vi "ScriptCommands.vi"(11 "Auton Routines":T1[](array[typedef])) -> ()   [LabVIEW 2013]
uses:
  Command Type.ctl
  <vilib>/Rock Robotics/WPI/DriverStation/DriverStationLCD/WPI_DriverStationLCDLCDLine.ctl
  Intake Actions.ctl
  <vilib>/Rock Robotics/WPI/RobotDrive/WPI_RobotDriveGetSetRefNum.vi
  Auto Pickup Global.vi
  Robot Global Data.vi
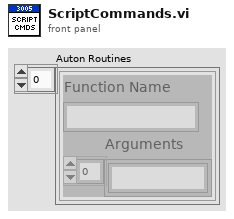
[diagram p1: front panel]
types:
  T1 = typedef "Command Type.ctl" = cluster{"Function Name":string, "Arguments":string[]}
  T2 = typedef "WPI_DriverStationLCDLCDLine.ctl" = enum16{"Main - Line 1", "User - Line 2", "User - Line 3", "User - Line 4", "User - Line 5", "User - Line 6"}
  T3 = typedef "Intake Actions.ctl" = enum16{"Extend", "Contain", "Motor Still", "Motor Outward", "Motor Inward", "Collect", "Pass", "Herd", "Contain Off", "Collect Delay Off", "Patea"}
  T4 = typedef "WPI_EncoderDevRef.ctl" = cluster{"DevStatus":errorcluster, "EncoderIndex":T5, "CounterIndex":T6, "DistancePerCount":dbl, "Decoding Type":T7}
  T5 = typedef "FPGA_EncoderIdx.ctl" = enum8{"Enc 0", "Enc 1", "Enc 2", "Enc 3", "Invalid"}
  T6 = typedef "FPGA_CounterCtrSystemIndex.ctl" = enum8{"Ctr 0", "Ctr 1", "Ctr 2", "Ctr 3", "Ctr 4", "Ctr 5", "Ctr 6", "Ctr 7", "Invalid"}
  T7 = typedef "WPI_EncoderType.ctl" = enum16{"1x", "2x", "4x"}
  T8 = typedef "WPI_RobotDriveDevRef.ctl" = cluster{"DevStatus":errorcluster, "Motors[]":T9[], "Square Inputs":bool, "Max Output":dbl, "Isochronous":bool}
  T9 = typedef "WPI_MotorControlDeviceRef.ctl" = cluster{"DeviceStatus":errorcluster, "Type":enum16{"PWM", "CAN"}, "PWM":cluster{"Digital Module":T10, "PWM Channel":T11, "DeadBand":T12}, "CAN":cluster{"Device Number":u8, "Control Mode":T13, "Semaphore":T14, "Max Vout":dbl}, "Invert":bool, "TransformRef":T15, "InvTransformRef":T15}
  T10 = typedef "FPGA_TypedefDigitalModule.ctl" = enum16{"Digital Module 1", "Digital Module 2"}
  T11 = typedef "FPGA_DIOPWMChannel.ctl" = enum8{"PWM 1", "PWM 2", "PWM 3", "PWM 4", "PWM 5", "PWM 6", "PWM 7", "PWM 8", "PWM 9", "PWM 10", "Invalid"}
  T12 = typedef "WPI_PWMDeadband.ctl" = cluster{"Name":string, "maxPositivePwm":i32, "minPositivePwm":i32, "centerPwm":i32, "maxNegativePwm":i32, "minNegativePwm":i32, "angularRange":u16}
  T13 = typedef "WPI_CANJaguar_ControlMode.ctl" = enum8{"Percent VBus", "Current", "Speed", "Position", "Voltage"}
  T14 = typedef "Semaphore RefNum" = refnum<k1>
  T15 = typedef "WPI_PWMTransform_ConPane.ctl" = refnum<vi>
  T16 = typedef "WPI_CounterDevRef.ctl" = cluster{"DevStatus":errorcluster, "CntIndex":T6}
  T17 = typedef "WPI_GyroDevRef.ctl" = cluster{"DevStatus":errorcluster, "Analog Module":T18, "Analog Channel":T19, "Offset":dbl, "Gain (VoltsPerDegree/Second)":dbl}
  T18 = typedef "FPGA_TypedefAnalogModule.ctl" = enum16{"Analog Module 1", "Analog Module 2"}
  T19 = typedef "FPGA_AIChannel.ctl" = enum8{"AI 1", "AI 2", "AI 3", "AI 4", "AI 5", "AI 6", "AI 7", "AI 8", "Invalid"}
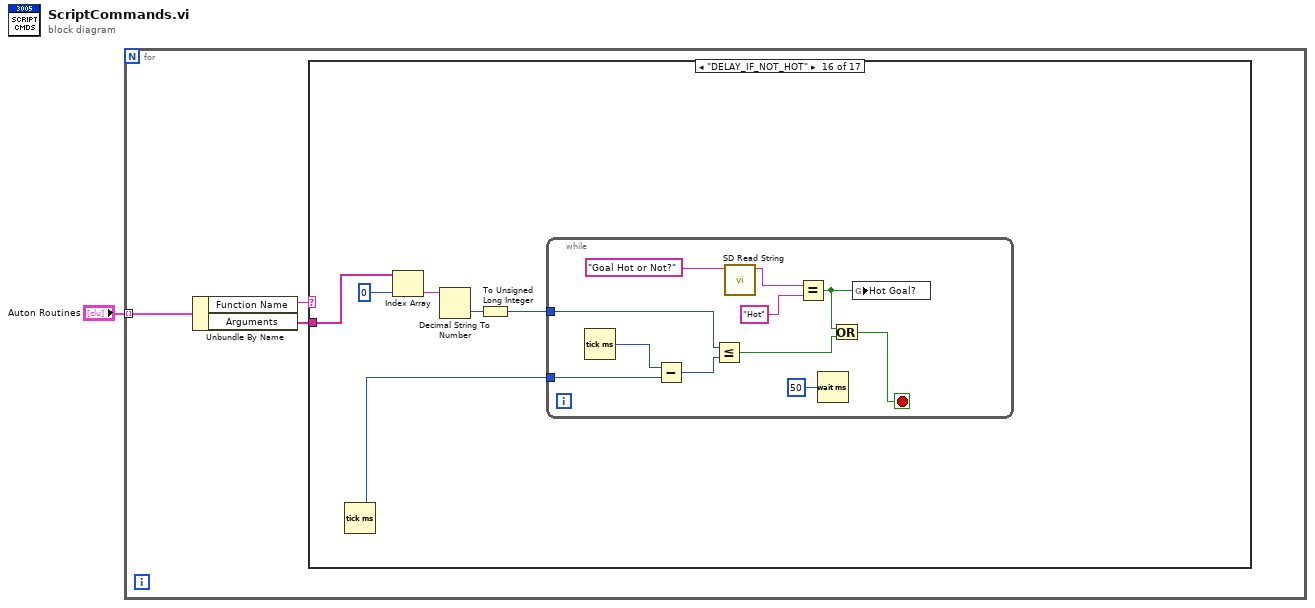
[diagram p0: block diagram]
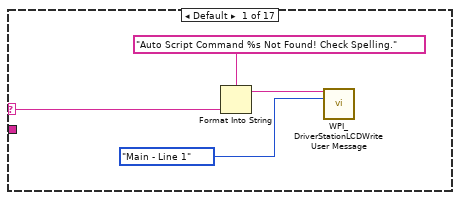
[diagram p2: hidden frame]
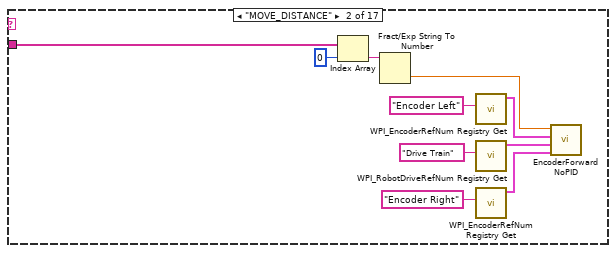
[diagram p3: hidden frame]
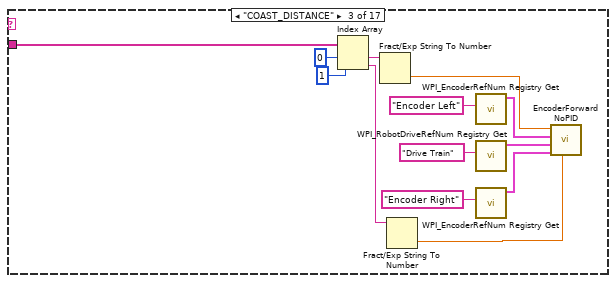
[diagram p4: hidden frame]
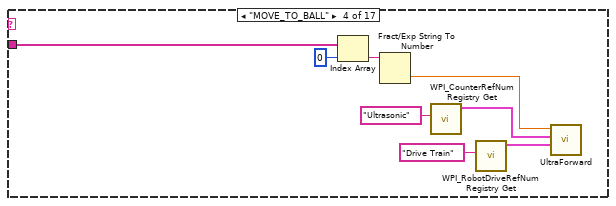
[diagram p5: hidden frame]
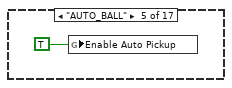
[diagram p6: hidden frame]
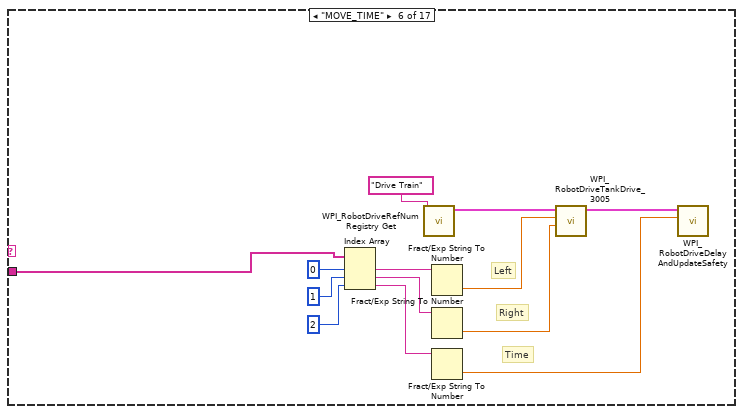
[diagram p7: hidden frame]
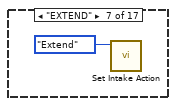
[diagram p8: hidden frame]
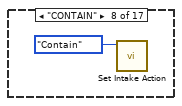
[diagram p9: hidden frame]
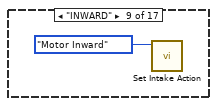
[diagram p10: hidden frame]
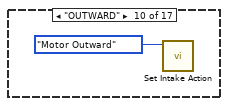
[diagram p11: hidden frame]
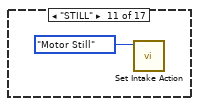
[diagram p12: hidden frame]
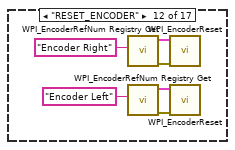
[diagram p13: hidden frame]
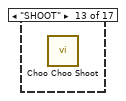
[diagram p14: hidden frame]
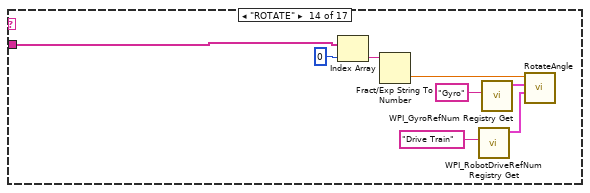
[diagram p15: hidden frame]
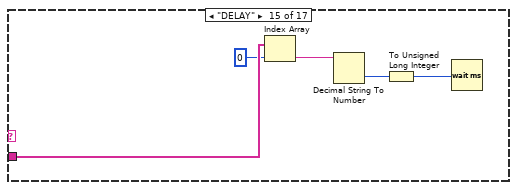
[diagram p16: hidden frame]
diagram:
  n1 = for {
    tunnel: "Auton Routines" -> [w4] mode=indexing
    n2 = Unbundle By Name(w4) -> ("Function Name"=w3:string, "Arguments"=w2:string[])
    n3 = case shown="\"DELAY_IF_NOT_HOT\"" w3 {
      selector: w3 -> [w8 _ _ _ _ _ _ _ _ _ _ _ _ _ _ _ _]
      tunnel: w2 -> [_ w18 w31 w39 _ w41 _ _ _ _ _ _ _ w72 w77 w80 _]
      frame Default {
        n4 = Format Into String(format string="Auto Script Command %s Not Found! Check Spelling.", w8) -> (resulting string=w6:string)  [unwired: 2 in, 1 out]
        n5 = call <vilib>:"WPI_DriverStationLCDWrite User Message.vi"("line text"=w6, "line"=WPI_DriverStationLCDLCDLine."Main - Line 1") -> ()  [unwired: 13 in, 1 out]
      }
      frame "MOVE_DISTANCE" {
        n6 = Index Array(array=w18, index=0) -> (element=w16:string)
        n7 = Fract/Exp String To Number(string=w16) -> (number=w9:dbl)  [unwired: 3 in, 1 out]
        n8 = call <vilib>:"WPI_EncoderRefNum Registry Get.vi"("refnum name"="Encoder Left") -> ("EncoderDevRef"=w10:T4)  [unwired: 9 in, 1 out]
        n9 = call <vilib>:"WPI_RobotDriveRefNum Registry Get.vi"("refnum name"="Drive Train") -> ("RobotDriveDevRef"=w14:T8)  [unwired: 1 in, 9 out]
        n10 = call <vilib>:"WPI_EncoderRefNum Registry Get.vi"("refnum name"="Encoder Right") -> ("EncoderDevRef"=w11:T4)  [unwired: 9 in, 1 out]
        n11 = call "EncoderForwardNoPID.vi"("EncoderDevRef 4"=w11, "RobotDriveDevRef"=w14, "EncoderDevRef"=w10, "Target"=w9) -> ()  [unwired: 5 in, 3 out]
      }
      frame "COAST_DISTANCE" {
        n12 = Index Array(array=w31, index #1=0 ("index"), index #2=1 ("index")) -> (element #1=w29:string, element #2=w20:string)
        n13 = Fract/Exp String To Number(string=w29) -> (number=w22:dbl)  [unwired: 3 in, 1 out]
        n14 = Fract/Exp String To Number(string=w20) -> (number=w21:dbl)  [unwired: 3 in, 1 out]
        n15 = call <vilib>:"WPI_EncoderRefNum Registry Get.vi"("refnum name"="Encoder Left") -> ("EncoderDevRef"=w23:T4)  [unwired: 9 in, 1 out]
        n16 = call <vilib>:"WPI_RobotDriveRefNum Registry Get.vi"("refnum name"="Drive Train") -> ("RobotDriveDevRef"=w27:T8)  [unwired: 1 in, 9 out]
        n17 = call <vilib>:"WPI_EncoderRefNum Registry Get.vi"("refnum name"="Encoder Right") -> ("EncoderDevRef"=w24:T4)  [unwired: 9 in, 1 out]
        n18 = call "EncoderForwardNoPID.vi"("Right axis value"=w21, "EncoderDevRef 4"=w24, "RobotDriveDevRef"=w27, "EncoderDevRef"=w23, "Target"=w22) -> ()  [unwired: 4 in, 3 out]
      }
      frame "MOVE_TO_BALL" {
        n19 = Index Array(array=w39, index=0) -> (element=w37:string)
        n20 = Fract/Exp String To Number(string=w37) -> (number=w34:dbl)  [unwired: 3 in, 1 out]
        n21 = call <vilib>:"WPI_CounterRefNum Registry Get.vi"("refnum name"="Ultrasonic") -> ("CounterDevRef"=w33:T16)  [unwired: 9 in, 1 out]
        n22 = call <vilib>:"WPI_RobotDriveRefNum Registry Get.vi"("refnum name"="Drive Train") -> ("RobotDriveDevRef"=w35:T8)  [unwired: 1 in, 9 out]
        n23 = call "UltraForward.vi"("RobotDriveDevRef"=w35, "CounterDevRef in"=w33, "Target"=w34) -> ()  [unwired: 8 in, 1 out]
      }
      frame "AUTO_BALL" {
        n24 = global write "Auto Pickup Global.vi" "Enable Auto Pickup"(TRUE ("Enable Auto Pickup")) -> ()
      }
      frame "MOVE_TIME" {
        # "Time"
        # "Right"
        # "Left"
        n25 = Index Array(array=w41, index #1=0 ("index"), index #2=1 ("index"), index #3=2 ("index")) -> (element #1=w47:string, element #2=w46:string, element #3=w45:string)
        n26 = call <vilib>:"WPI_RobotDriveRefNum Registry Get.vi"("refnum name"="Drive Train") -> ("RobotDriveDevRef"=w51:T8)  [unwired: 1 in, 9 out]
        n27 = Fract/Exp String To Number(string=w47) -> (number=w44:dbl)  [unwired: 3 in, 1 out]
        n28 = Fract/Exp String To Number(string=w46) -> (number=w43:dbl)  [unwired: 3 in, 1 out]
        n29 = Fract/Exp String To Number(string=w45) -> (number=w42:dbl)  [unwired: 3 in, 1 out]
        n30 = call <vilib>:"WPI_RobotDriveTankDrive_3005.vi"("Right axis value"=w43, "Left axis value"=w44, "RobotDriveDevRef"=w51) -> ("RobotDriveDevRef"=w53:T8)  [unwired: 6 in, 2 out]
        n31 = call <vilib>:"WPI_RobotDriveDelayAndUpdateSafety.vi"("Delay (s)"=w42, "RobotDriveDevRef"=w53) -> ()  [unwired: 8 in, 2 out]
      }
      frame "EXTEND" {
        n32 = call "Set Intake Action.vi"("Action"=Intake_Actions."Extend") -> ()  [unwired: 10 in, 1 out]
      }
      frame "CONTAIN" {
        n33 = call "Set Intake Action.vi"("Action"=Intake_Actions."Contain") -> ()  [unwired: 10 in, 1 out]
      }
      frame "INWARD" {
        n34 = call "Set Intake Action.vi"("Action"=Intake_Actions."Motor Inward") -> ()  [unwired: 10 in, 1 out]
      }
      frame "OUTWARD" {
        n35 = call "Set Intake Action.vi"("Action"=Intake_Actions."Motor Outward") -> ()  [unwired: 10 in, 1 out]
      }
      frame "STILL" {
        n36 = call "Set Intake Action.vi"("Action"=Intake_Actions."Motor Still") -> ()  [unwired: 10 in, 1 out]
      }
      frame "RESET_ENCODER" {
        n37 = call <vilib>:"WPI_EncoderRefNum Registry Get.vi"("refnum name"="Encoder Right") -> ("error out"=w64:errorcluster, "EncoderDevRef"=w63:T4)  [unwired: 9 in]
        n38 = call <vilib>:"WPI_EncoderRefNum Registry Get.vi"("refnum name"="Encoder Left") -> ("error out"=w59:errorcluster, "EncoderDevRef"=w60:T4)  [unwired: 9 in]
        n39 = call <vilib>:"WPI_EncoderReset.vi"("error in (no error)"=w64, "EncoderDevRef"=w63) -> ()  [unwired: 8 in, 2 out]
        n40 = call <vilib>:"WPI_EncoderReset.vi"("error in (no error)"=w59, "EncoderDevRef"=w60) -> ()  [unwired: 8 in, 2 out]
      }
      frame "SHOOT" {
        n41 = call "Choo Choo Shoot.vi"() -> ()  [unwired: 11 in, 1 out]
      }
      frame "ROTATE" {
        n42 = Index Array(array=w72, index=0) -> (element=w70:string)
        n43 = Fract/Exp String To Number(string=w70) -> (number=w65:dbl)  [unwired: 3 in, 1 out]
        n44 = call <vilib>:"WPI_RobotDriveRefNum Registry Get.vi"("refnum name"="Drive Train") -> ("RobotDriveDevRef"=w66:T8)  [unwired: 1 in, 9 out]
        n45 = call <vilib>:"WPI_GyroRefNum Registry Get.vi"("refnum name"="Gyro") -> ("GyroDevRef"=w69:T17)  [unwired: 9 in, 1 out]
        n46 = call "RotateAngle.vi"("RobotDriveDevRef"=w66, "GyroDevRef"=w69, "Target"=w65) -> ()  [unwired: 7 in, 2 out]
      }
      frame "DELAY" {
        n47 = Index Array(array=w77, index=0) -> (element=w75:string)
        n48 = Decimal String To Number(string=w75) -> (number=w74:i32)  [unwired: 2 in, 1 out]
        n49 = To Unsigned Long Integer(number=w74) -> (unsigned 32bit integer=w73:u32)
        n50 = Wait (ms)(milliseconds to wait=w73) -> ()  [unwired: 1 out]
      }
      frame "DELAY_IF_NOT_HOT" {
        n51 = Tick Count (ms)() -> (millisecond timer value=w79:u32)
        n52 = Index Array(array=w80, index=0) -> (element=w82:string)
        n53 = Decimal String To Number(string=w82) -> (number=w81:i32)  [unwired: 2 in, 1 out]
        n54 = To Unsigned Long Integer(number=w81) -> (unsigned 32bit integer=w78:u32)
        n55 = while {
          tunnel: w79 -> [w93]
          tunnel: w78 -> [w88]
          stop <- w85 stop-if-true
          n56 = Tick Count (ms)() -> (millisecond timer value=w92:u32)
          n57 = Subtract(x=w92, y=w93) -> (x-y=w91:u32)
          n58 = Less Or Equal?(x=w88, y=w91) -> (x <= y?=w90:bool)
          n59 = call <vilib>:"SD Read String.vi"("Name"="Goal Hot or Not?") -> ("String"=w87:string)  [unwired: 8 in, 2 out]
          n60 = Equal?(x=w87, y="Hot") -> (x = y?=w84:bool)
          n61 = Wait (ms)(milliseconds to wait=u32 50) -> ()  [unwired: 1 out]
          n62 = Or(x=w84, y=w90) -> (x .or. y?=w85:bool)
          n63 = global write "Robot Global Data.vi" "Hot Goal?"(w84) -> ()
        }
      }
      frame "STOP" {
      }
    }
  }
